vi "Test_Class Load.vi"() -> ()   [LabVIEW 2019]
uses:
  ClassLoader.lvlib
panel:
  out "Loaded Class":refnum<class>
  out "Success?":bool
  out "error out":errorcluster
  in  "error in (no error)":errorcluster
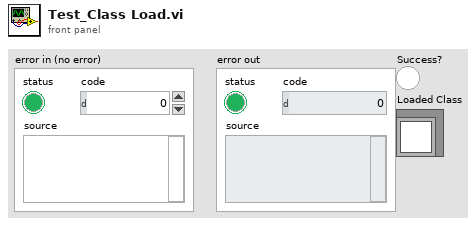
[diagram p1: front panel]
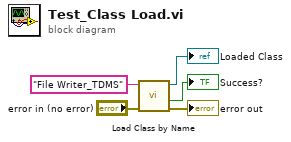
[diagram p0: block diagram]
diagram:
  n1 = call "Load Class by Name.vi"("error in (no error)"="error in (no error)", "Base Class Name"="File Writer_TDMS") -> ("error out"=→"error out":errorcluster, "Load and Type Success?"=→"Success?":bool, "Loaded Class"=→"Loaded Class":refnum<class>)  [unwired: 6 in, 1 out]
